vi "GUI - TDMS (V2.00).vi"(0 "Time Data IN":refnum<class "GSwFormDSP.lvclass">, 5 "error in (no error)":errorcluster, 7 "Application Name":string="GSwForm", 9 "State Queue":string[](array[string])=["SC >>> Initialize"], 11 "TDMS - READ":path, 13 "TDMS - WRITE":path) -> (12 "Loaded File":path, 14 "SubVI Time Data DUP":refnum<class "GSwFormDSP.lvclass">, 19 "error out":errorcluster)   [LabVIEW 2020, in "TDMS.lvclass"]
uses:
  TDMS.lvclass
  API/GSwFormDSP_class/GSwFormDSP.lvclass
  <vilib>/Utility/sysdir.llb/System Directory Type.ctl
  C:/Users/fcharett/docsWork/coding/20openSourceSPWB/API/Generic Utilities_class/Generic Utilities.lvclass
  <userlib>/_OpenG.lib/array/array.llb/Filter 1D Array with Scalar (String)__ogtk.vi
  <userlib>/_OpenG.lib/array/array.llb/Remove Duplicates from 1D Array (String)__ogtk.vi
  <vilib>/addons/_AddQ/G#Object/G#Object.lvclass
  API/Generic Utilities_class/Generic Utilities.lvclass
panel:
  in  "Task":T1(tab)
  in  "Import Signals":bool
  in  "Select Signal to Import":i32[](listbox)
  in  "Exit":bool
  in  "Downsampling":enum16{"None", "By 10", "By 100", "By 1000"}(ring)=enum."By 10"
  out "Base Folder":path
  out "Number of TDMS Files":i32
  in  "Select Base Folder":bool
  in  "Defrag ALL Files":bool
  in  "Channel List":i32[](listbox)
  in  "Refresh Signal Names":bool
  in  "Select Multi Files":bool
  out "File List":path[](array[path])
  out "group/channel names":string[][](array[string])
  out "All T0":timestamp[](array[timestamp])
  out "Valid T0":bool
  out "Time Data":waveform(dbl)[](graph)
  in  "READ - Select TDMS File":bool
  in  "WRITE - Select Wave File":bool
  out "State History":string[](array[string])
  out "State Index":i32
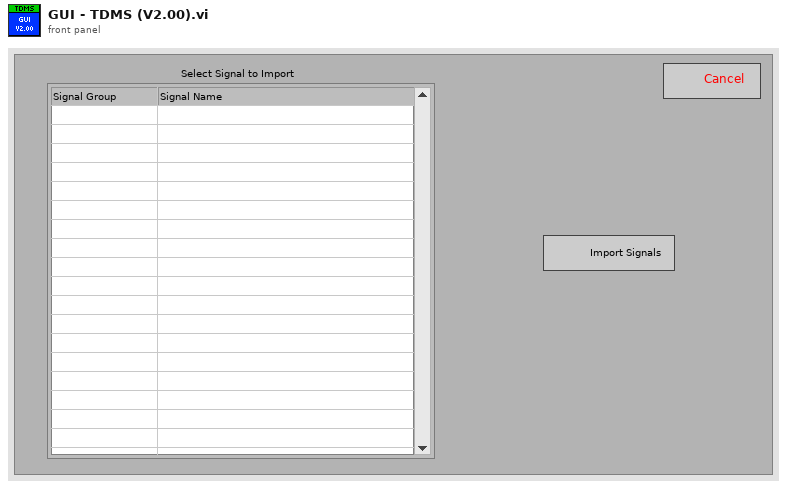
[diagram p1: front panel]
types:
  T1 = enum32{"TDMS Select Signal", "TDMS Folder", "Multi TDMS Files", "TDMS", "Settings"}
  T2 = enum32{"Invalid", "Standard", "Closed", "Hidden", "Minimized", "Maximized"}
  T3 = typedef "System Directory Type.ctl" = i32
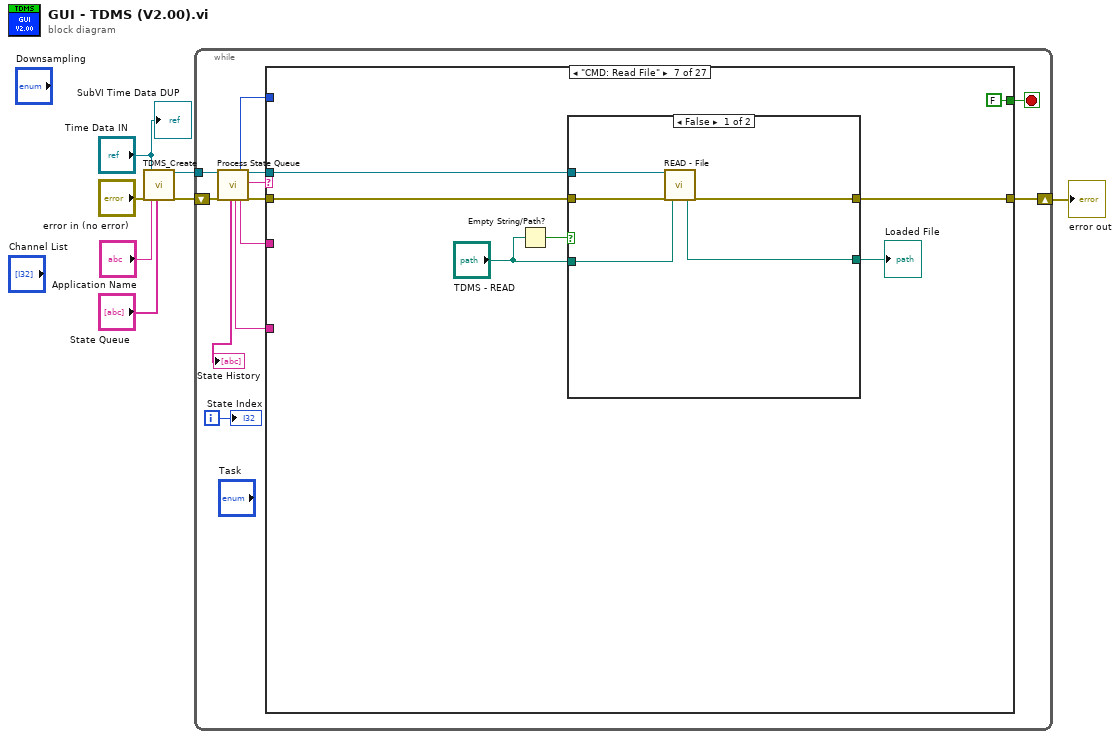
[diagram p0: block diagram]
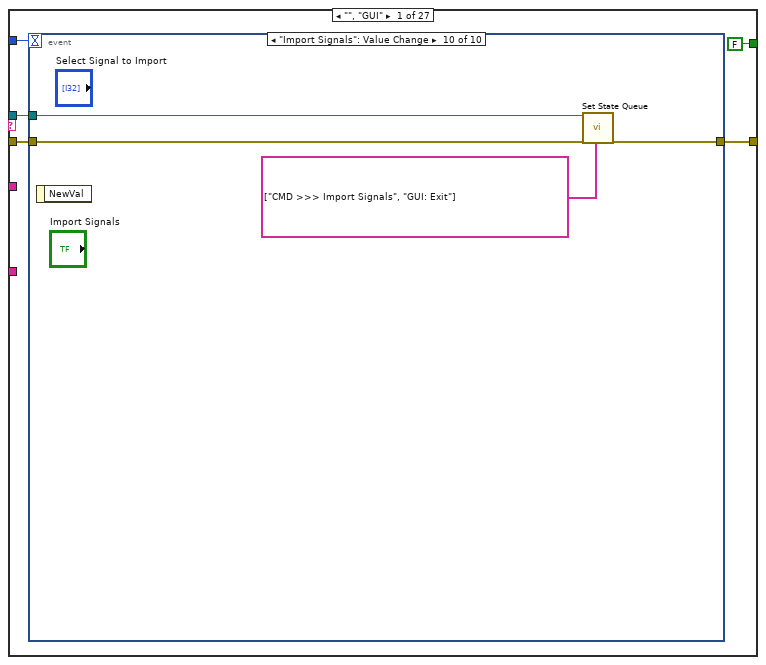
[diagram p2: hidden frame]
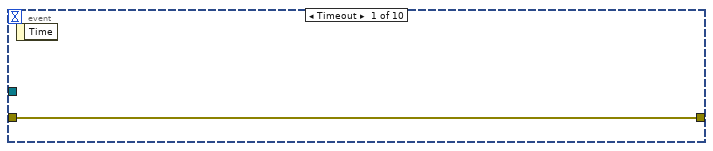
[diagram p3: hidden frame]
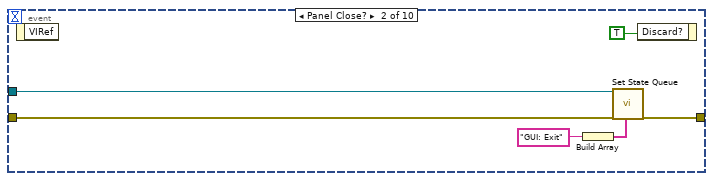
[diagram p4: hidden frame]
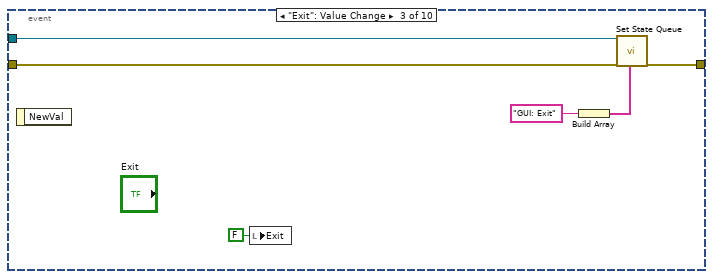
[diagram p5: hidden frame]
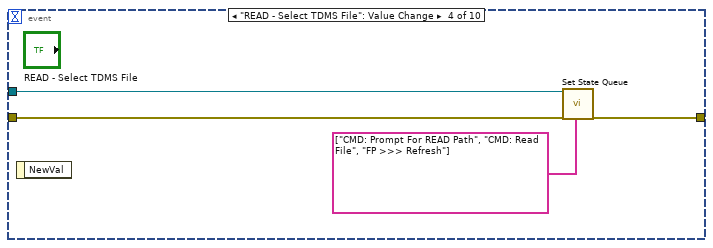
[diagram p6: hidden frame]
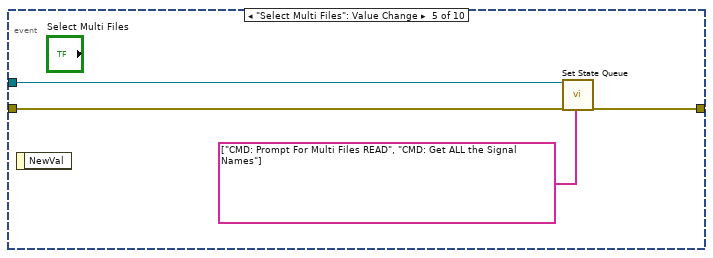
[diagram p7: hidden frame]
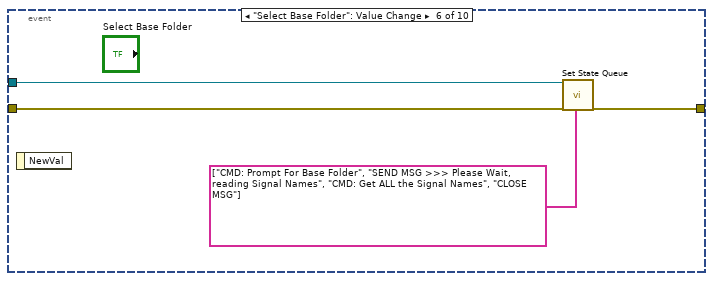
[diagram p8: hidden frame]
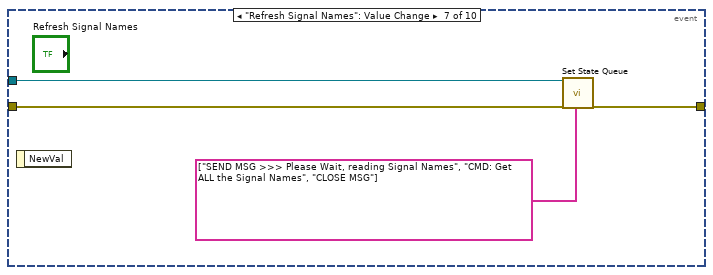
[diagram p9: hidden frame]
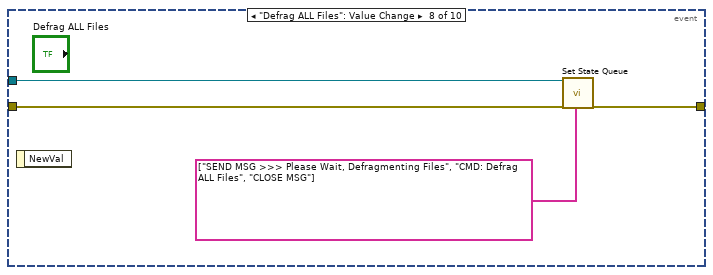
[diagram p10: hidden frame]
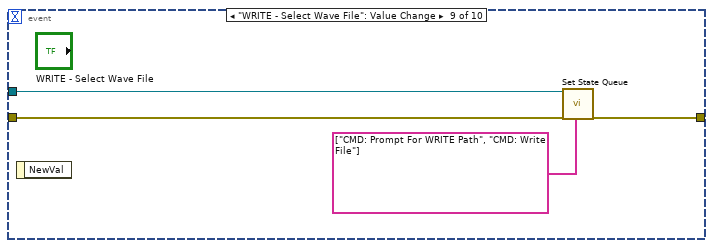
[diagram p11: hidden frame]
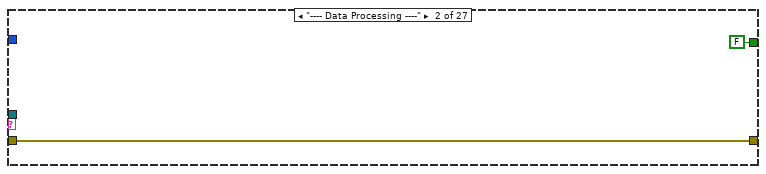
[diagram p12: hidden frame]
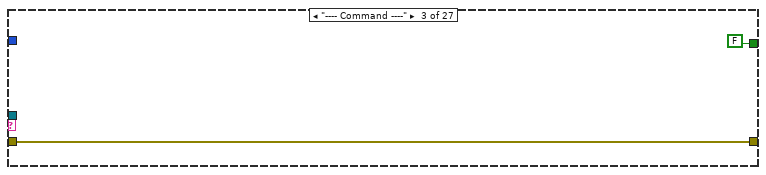
[diagram p13: hidden frame]
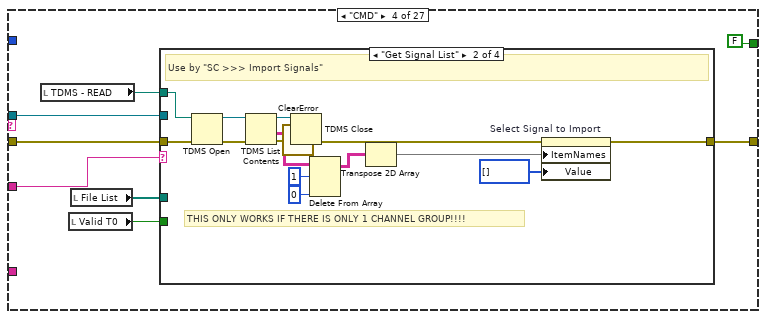
[diagram p14: hidden frame]
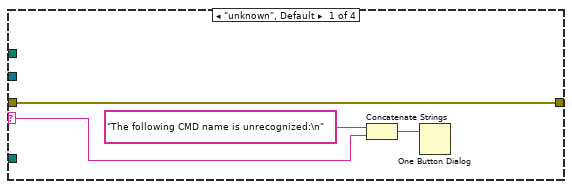
[diagram p15: hidden frame]
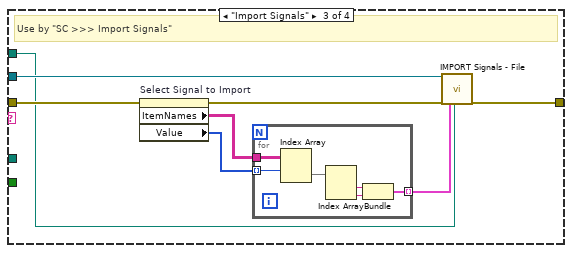
[diagram p16: hidden frame]
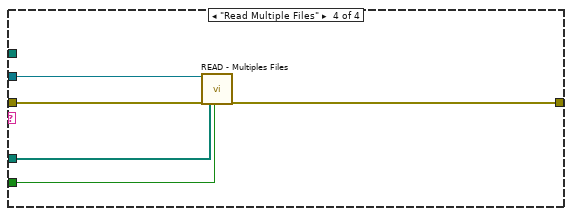
[diagram p17: hidden frame]
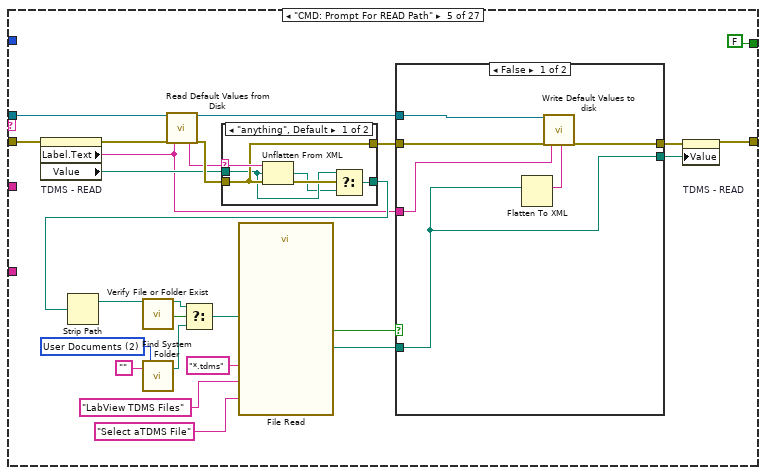
[diagram p18: hidden frame]
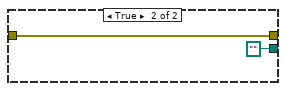
[diagram p19: hidden frame]
diagram:
  n1 = call "TDMS_Create.vi"("error in (no error)"="error in (no error)", "Time Data"="Time Data IN", "Application Name"="Application Name", "State Queue"="State Queue") -> ("reference out"=w7:refnum<class "TDMS.lvclass">, "error out"=w6:errorcluster)  [unwired: 14 in]
  n2 = while {
    shift-right: [w10] -> w2
    shift-left: w6 -> [w16]
    tunnel: w7 -> [w17]
    i -> [w18]
    stop <- w19 stop-if-true
    n3 = call "Process State Queue.vi"("reference in"=w17, "error in (no error)"=w16) -> ("State History"=→"State History":string[], "Additional Options"=w8:string, "Timeout"=w15:i32, "State Option"=w12:string, "reference out"=w14:refnum<class "TDMS.lvclass">, "Current State"=w13:string, "error out"=w11:errorcluster)  [unwired: 10 in, 1 out]
    n4 = case shown="\"CMD: Read File\"" w13 {
      selector: w13 -> [_ _ _ _ _ _ _ _ _ _ _ _ _ _ _ _ _ _ _ _ _ _ _ w614 _ _ _]
      tunnel: w14 -> [w22 _ _ w73 w140 w182 w205 w218 w250 w298 _ _ _ w404 _ w421 w476 _ w517 w538 w571 w596 _ _ _ _ w622]
      tunnel: [FALSE FALSE FALSE FALSE FALSE FALSE FALSE FALSE FALSE FALSE FALSE FALSE FALSE FALSE FALSE FALSE FALSE FALSE FALSE TRUE FALSE FALSE FALSE FALSE FALSE FALSE TRUE] -> w19
      tunnel: w15 -> [w23 _ _ _ _ _ _ _ _ _ _ _ _ _ _ _ _ _ _ _ _ _ _ _ _ _ _]
      tunnel: w12 -> [_ _ _ w76 _ _ _ _ _ _ _ _ _ w400 _ w422 w473 _ _ _ w580 _ _ _ _ _ _]
      tunnel: w11 -> [w21 w66 w68 w75 w139 w181 w204 w217 w249 w297 w339 w392 w397 w403 w416 w419 w475 w502 w514 w535 w570 w597 w610 w612 w617 w620 w623]
      tunnel: [w20 w66 w68 w74 w123 w165 w203 w216 w233 w283 w334 w389 w397 w402 w416 w420 w474 w502 w509 w534 w568 w593 w610 w612 errorcluster {"status"=FALSE, "code"=0, "source"=""} ("error out") w620 w624] -> w10
      tunnel: w8 -> [_ _ _ _ _ _ _ _ _ _ _ _ _ w399 _ w418 _ _ _ _ _ _ _ _ _ _ _]
      frame "", "GUI" {
        n5 = event shown="[9] \"Import Signals\": Value Change" {
          selector: _ -> [_ _ _ _ _ _ _ _ _ _]
          dyn-events: _ -> [_ _ _ _ _ _ _ _ _ _]
          timeout: w23 -> [_ _ _ _ _ _ _ _ _ _]
          tunnel: w22 -> [_ w29 w35 w40 w44 w48 w52 w56 w60 w64]
          tunnel: w21 -> [w25 w28 w33 w39 w43 w47 w51 w55 w59 w63]
          tunnel: [w25 w27 w34 w41 w45 w49 w53 w57 w61 w65] -> w20
          event Timeout {
            n6 = event-data() -> ()  [unwired: 1 in, 1 out]
          }
          event Panel Close? {
            n7 = event-data() -> ()  [unwired: 1 in, 1 out]
            n8 = Build Array("GUI: Exit") -> (w26:string[])
            n9 = call "Set State Queue.vi"("reference in"=w29, "error in (no error)"=w28, "State Queue"=w26) -> ("error out"=w27:errorcluster)  [unwired: 15 in, 1 out]
            n10 = event-data("Discard?"=TRUE) -> ()  [unwired: 1 in, 1 out]
          }
          event "Exit": Value Change {
            n11 = event-data() -> ()  [unwired: 1 in, 1 out]
            n12 = local write "Exit"(FALSE ("Exit")) -> ()
            n13 = Build Array("GUI: Exit") -> (w32:string[])
            n14 = call "Set State Queue.vi"("reference in"=w35, "error in (no error)"=w33, "State Queue"=w32) -> ("error out"=w34:errorcluster)  [unwired: 15 in, 1 out]
          }
          event "READ - Select TDMS File": Value Change {
            n15 = event-data() -> ()  [unwired: 1 in, 1 out]
            n16 = call "Set State Queue.vi"("reference in"=w40, "error in (no error)"=w39, "State Queue"=string[] ["CMD: Prompt For READ Path", "CMD: Read File", "FP >>> Refresh"]) -> ("error out"=w41:errorcluster)  [unwired: 15 in, 1 out]
          }
          event "Select Multi Files": Value Change {
            n17 = event-data() -> ()  [unwired: 1 in, 1 out]
            n18 = call "Set State Queue.vi"("reference in"=w44, "error in (no error)"=w43, "State Queue"=string[] ["CMD: Prompt For Multi Files READ", "CMD: Get ALL the Signal Names"]) -> ("error out"=w45:errorcluster)  [unwired: 15 in, 1 out]
          }
          event "Select Base Folder": Value Change {
            n19 = event-data() -> ()  [unwired: 1 in, 1 out]
            n20 = call "Set State Queue.vi"("reference in"=w48, "error in (no error)"=w47, "State Queue"=string[] ["CMD: Prompt For Base Folder", "SEND MSG >>> Please Wait, reading Signal Names", "CMD: Get ALL the Signal Names", "CLOSE MSG"]) -> ("error out"=w49:errorcluster)  [unwired: 15 in, 1 out]
          }
          event "Refresh Signal Names": Value Change {
            n21 = event-data() -> ()  [unwired: 1 in, 1 out]
            n22 = call "Set State Queue.vi"("reference in"=w52, "error in (no error)"=w51, "State Queue"=string[] ["SEND MSG >>> Please Wait, reading Signal Names", "CMD: Get ALL the Signal Names", "CLOSE MSG"]) -> ("error out"=w53:errorcluster)  [unwired: 15 in, 1 out]
          }
          event "Defrag ALL Files": Value Change {
            n23 = event-data() -> ()  [unwired: 1 in, 1 out]
            n24 = call "Set State Queue.vi"("reference in"=w56, "error in (no error)"=w55, "State Queue"=string[] ["SEND MSG >>> Please Wait, Defragmenting Files", "CMD: Defrag ALL Files", "CLOSE MSG"]) -> ("error out"=w57:errorcluster)  [unwired: 15 in, 1 out]
          }
          event "WRITE - Select Wave File": Value Change {
            n25 = event-data() -> ()  [unwired: 1 in, 1 out]
            n26 = call "Set State Queue.vi"("reference in"=w60, "error in (no error)"=w59, "State Queue"=string[] ["CMD: Prompt For WRITE Path", "CMD: Write File"]) -> ("error out"=w61:errorcluster)  [unwired: 15 in, 1 out]
          }
          event "Import Signals": Value Change {
            n27 = event-data() -> ()  [unwired: 1 in, 1 out]
            n28 = call "Set State Queue.vi"("reference in"=w64, "error in (no error)"=w63, "State Queue"=string[] ["CMD >>> Import Signals", "GUI: Exit"]) -> ("error out"=w65:errorcluster)  [unwired: 15 in, 1 out]
          }
        }
      }
      frame "---- Data Processing ----" {
      }
      frame "---- Command ----" {
      }
      frame "CMD" {
        n29 = local read "TDMS - READ"() -> (w72:path)
        n30 = local read "Valid T0"() -> (w70:bool)
        n31 = local read "File List"() -> (w71:path[])
        n32 = case shown="\"Get Signal List\"" w76 {
          selector: w76 -> [w79 _ _ _]
          tunnel: w75 -> [w78 w94 w102 w114]
          tunnel: [w78 w90 w103 w113] -> w74
          tunnel: w73 -> [_ _ w104 w115]
          tunnel: w72 -> [_ w83 w99 _]
          tunnel: w71 -> [_ _ _ w112]
          tunnel: w70 -> [_ _ _ w111]
          frame "unknown", Default {
            n33 = Concatenate Strings("The following CMD name is unrecognized:\n", w79) -> (w80:string)
            n34 = One Button Dialog(message=w80) -> ()  [unwired: 1 in, 1 out]
          }
          frame "Get Signal List" {
            # "THIS ONLY WORKS IF THERE IS ONLY 1 CHANNEL GROUP!!!!"
            # "Use by \"SC >>> Import Signals\""
            n35 = TDMS Open(8:w94, 11:w83) -> (0:w96:errorcluster, 3:w95:refnum<k34>)  [unwired: 5 in]
            n36 = TDMS List Contents(4:w96, 7:w95) -> (0:w82:errorcluster, 1:w88:string[][], 3:w92:refnum<k34>)  [unwired: 1 in, 1 out]
            n37 = call <vilib>:"ClearError.vi"("error in (no error)"=w82) -> ("error out"=w93:errorcluster)
            n38 = TDMS Close(8:w93, 11:w92) -> (0:w91:errorcluster)  [unwired: 1 out]
            n39 = Delete From Array(array=w88, length=1, index (col)=0 ("disabled index (col)")) -> (array with subset deleted=w85:string[][])  [unwired: 1 in, 1 out]
            n40 = Transpose 2D Array(2D array=w85) -> (transposed array=w89:string[][])
            n41 = property on="Select Signal to Import" class="MCListbox (strict)"(error in=w91, "ItemNames"=w89, "Value"=i32[] [] ("Select Signal to Import")) -> (error out=w90:errorcluster)  [unwired: 1 in, 1 out]
          }
          frame "Import Signals" {
            # "Use by \"SC >>> Import Signals\""
            n42 = property on="Select Signal to Import" class="MCListbox (strict)"(error in=w102) -> (error out=w98:errorcluster, "ItemNames"=w101:string[][], "Value"=w100:i32[])  [unwired: 1 in, 1 out]
            n43 = for {
              tunnel: w101 -> [w110]
              tunnel: w100 -> [w109] mode=indexing
              tunnel: [w105] -> w97 mode=indexing
              n44 = Index Array(array=w110, index (row)=w109) -> (element=w108:string[])  [unwired: 1 in]
              n45 = Index Array(array=w108) -> (element #1=w106:string, element #2=w107:string)  [unwired: 2 in]
              n46 = Bundle(w106, w107) -> (w105:cluster{string, string})  [unwired: 1 in]
            }
            n47 = call "IMPORT Signals - File.vi"("reference in"=w104, "error in (no error)"=w98, "Grp/Sig Names"=w97, "TDMS Path - READ"=w99) -> ("error out"=w103:errorcluster)  [unwired: 14 in, 1 out]
          }
          frame "Read Multiple Files" {
            n48 = call "READ - Multiples Files.vi"("reference in"=w115, "error in (no error)"=w114, "File List"=w112, "Valid T0"=w111) -> ("error out"=w113:errorcluster)  [unwired: 14 in, 1 out]
          }
        }
      }
      frame "CMD: Prompt For READ Path" {
        w130 = T3 2 items=["User Home"=0, "User Desktop"=1, "User Documents"=2, "User Application Data"=3, "User Preferences"=4, "User Temporary"=5, "Public Documents"=6, "Public Application Data"=7, "Public Preferences"=8, "Public Cache"=13, "System Core Libraries"=9, "System Installed Libraries"=10, "Application Files"=11, "Boot Volume Root"=12] ("system directory type")
        n49 = property on="TDMS - READ" class="Path"(error in=w139) -> (error out=w138:errorcluster, "Label.Text"=w118:string, "Value"=w136:path)  [unwired: 1 in, 1 out]
        n50 = call "Find System Folder.vi"("Application Name"="", "system directory type"=w130) -> ("System Folder"=w129:path)  [unwired: 16 in, 1 out]
        n51 = call-dynamic "Read Default Values from Disk.vi"("reference in"=w140, "error in (no error)"=w138, "Control Label"=w118) -> ("Value (XML String)"=w116:string, "reference out"=w119:refnum<class "TDMS.lvclass">, "error out"=w137:errorcluster)  [unwired: 14 in]
        n52 = case shown="\"anything\", Default" w116 {
          selector: w116 -> [w155 _]
          tunnel: [w150 w157] -> w135
          tunnel: w136 -> [w152 w157]
          tunnel: w137 -> [w153 w156]
          tunnel: [w153 w156] -> w121
          frame "anything", Default {
            n53 = Unflatten From XML(xml string=w155, type=w152, error in (no error)=w153) -> (value=w151:path, error out=w154:errorcluster)
            n54 = Select(t=w152, s=w154, f=w151) -> (s? t:f=w150:path)
          }
          frame "" {
            # "Either the file was not found or there was some error"
          }
        }
        n55 = Strip Path(path=w135) -> (stripped path=w134:path)  [unwired: 1 out]
        n56 = call "Verify File or Folder Exist.vi"("path"=w134) -> ("dup path"=w132:path, "file or folder exists?"=w133:bool)  [unwired: 16 in, 1 out]
        n57 = Select(t=w132, s=w133, f=w129) -> (s? t:f=w131:path)
        n58 = call "File Read"("start path"=w131, "button label"="Select aTDMS File", "pattern (all files)"="*.tdms", "pattern label"="LabView TDMS Files") -> ("selected path"=w117:path, "cancelled"=w124:bool)  [unwired: 8 in, 2 out]
        n59 = case shown="False" w124 {
          tunnel: [w143 w149] -> w122
          tunnel: w121 -> [w144 w149]
          tunnel: [w142 path ""] -> w120
          tunnel: w119 -> [w146 _]
          tunnel: w118 -> [w145 _]
          tunnel: w117 -> [w142 _]
          frame False {
            n60 = Flatten To XML(6:w142) -> (2:w147:string)
            n61 = call-dynamic "Write Default Values to disk.vi"("reference in"=w146, "error in (no error)"=w144, "Control Label"=w145, "Value (XML String)"=w147) -> ("error out"=w143:errorcluster)  [unwired: 14 in, 1 out]
          }
          frame True {
          }
        }
        n62 = property on="TDMS - READ" class="Path"(error in=w122, "Value"=w120) -> (error out=w123:errorcluster)  [unwired: 1 in, 1 out]
      }
      frame "CMD: Prompt For WRITE Path" {
        w172 = T3 2 items=["User Home"=0, "User Desktop"=1, "User Documents"=2, "User Application Data"=3, "User Preferences"=4, "User Temporary"=5, "Public Documents"=6, "Public Application Data"=7, "Public Preferences"=8, "Public Cache"=13, "System Core Libraries"=9, "System Installed Libraries"=10, "Application Files"=11, "Boot Volume Root"=12] ("system directory type")
        n63 = property on="TDMS - WRITE" class="Path"(error in=w181) -> (error out=w180:errorcluster, "Label.Text"=w160:string, "Value"=w178:path)  [unwired: 1 in, 1 out]
        n64 = call "Find System Folder.vi"("Application Name"="", "system directory type"=w172) -> ("System Folder"=w171:path)  [unwired: 16 in, 1 out]
        n65 = call-dynamic "Read Default Values from Disk.vi"("reference in"=w182, "error in (no error)"=w180, "Control Label"=w160) -> ("Value (XML String)"=w158:string, "reference out"=w161:refnum<class "TDMS.lvclass">, "error out"=w179:errorcluster)  [unwired: 14 in]
        n66 = case shown="\"anything\", Default" w158 {
          selector: w158 -> [w197 _]
          tunnel: [w192 w199] -> w177
          tunnel: w178 -> [w194 w199]
          tunnel: w179 -> [w195 w198]
          tunnel: [w195 w198] -> w163
          frame "anything", Default {
            n67 = Unflatten From XML(xml string=w197, type=w194, error in (no error)=w195) -> (value=w193:path, error out=w196:errorcluster)
            n68 = Select(t=w194, s=w196, f=w193) -> (s? t:f=w192:path)
          }
          frame "" {
            # "Either the file was not found or there was some error"
          }
        }
        n69 = Strip Path(path=w177) -> (stripped path=w176:path)  [unwired: 1 out]
        n70 = call "Verify File or Folder Exist.vi"("path"=w176) -> ("dup path"=w174:path, "file or folder exists?"=w175:bool)  [unwired: 16 in, 1 out]
        n71 = Select(t=w174, s=w175, f=w171) -> (s? t:f=w173:path)
        n72 = call "File Write"("start path"=w173, "button label"="Select aTDMS File", "pattern (all files)"="*.tdms", "pattern label"="LabView TDMS Files") -> ("selected path"=w159:path, "cancelled"=w166:bool)  [unwired: 8 in, 2 out]
        n73 = case shown="False" w166 {
          tunnel: [w185 w191] -> w164
          tunnel: w163 -> [w186 w191]
          tunnel: [w184 path ""] -> w162
          tunnel: w161 -> [w188 _]
          tunnel: w160 -> [w187 _]
          tunnel: w159 -> [w184 _]
          frame False {
            n74 = Flatten To XML(6:w184) -> (2:w189:string)
            n75 = call-dynamic "Write Default Values to disk.vi"("reference in"=w188, "error in (no error)"=w186, "Control Label"=w187, "Value (XML String)"=w189) -> ("error out"=w185:errorcluster)  [unwired: 14 in, 1 out]
          }
          frame True {
          }
        }
        n76 = property on="TDMS - WRITE" class="Path"(error in=w164, "Value"=w162) -> (error out=w165:errorcluster)  [unwired: 1 in, 1 out]
      }
      frame "CMD: Read File" {
        n77 = Empty String/Path?(string/path="TDMS - READ") -> (empty?=w202:bool)
        n78 = case shown="False" w202 {
          tunnel: w205 -> [w211 _]
          tunnel: w204 -> [w210 w213]
          tunnel: [w208 w213] -> w203
          tunnel: "TDMS - READ" -> [w209 _]
          tunnel: [w207 path ""] -> w200
          frame False {
            n79 = call "READ - File.vi"("reference in"=w211, "error in (no error)"=w210, "TDMS Path - READ"=w209) -> ("File Loaded"=w207:path, "error out"=w208:errorcluster)  [unwired: 14 in, 1 out]
          }
          frame True {
            # "User cancelled, so do nothing!"
          }
        }
        "Loaded File" <- w200
      }
      frame "CMD: Write File" {
        n80 = Empty String/Path?(string/path="TDMS - WRITE") -> (empty?=w215:bool)
        n81 = case shown="False" w215 {
          tunnel: w218 -> [w223 _]
          tunnel: w217 -> [w222 w224]
          tunnel: [w220 w224] -> w216
          tunnel: "TDMS - WRITE" -> [w221 _]
          frame False {
            n82 = call "WRITE - File.vi"("reference in"=w223, "error in (no error)"=w222, "TDMS Path - WRITE"=w221) -> ("error out"=w220:errorcluster)  [unwired: 15 in, 1 out]
          }
          frame True {
            # "User cancelled, so do nothing!"
          }
        }
      }
      frame "CMD: Prompt For Multi Files READ" {
        w240 = T3 2 items=["User Home"=0, "User Desktop"=1, "User Documents"=2, "User Application Data"=3, "User Preferences"=4, "User Temporary"=5, "Public Documents"=6, "Public Application Data"=7, "Public Preferences"=8, "Public Cache"=13, "System Core Libraries"=9, "System Installed Libraries"=10, "Application Files"=11, "Boot Volume Root"=12] ("system directory type")
        n83 = property on="TDMS - READ" class="Path"(error in=w249) -> (error out=w248:errorcluster, "Label.Text"=w228:string, "Value"=w246:path)  [unwired: 1 in, 1 out]
        n84 = call "Find System Folder.vi"("Application Name"="", "system directory type"=w240) -> ("System Folder"=w239:path)  [unwired: 16 in, 1 out]
        n85 = call-dynamic "Read Default Values from Disk.vi"("reference in"=w250, "error in (no error)"=w248, "Control Label"=w228) -> ("Value (XML String)"=w225:string, "reference out"=w229:refnum<class "TDMS.lvclass">, "error out"=w247:errorcluster)  [unwired: 14 in]
        n86 = case shown="\"anything\", Default" w225 {
          selector: w225 -> [w271 _]
          tunnel: [w266 w273] -> w245
          tunnel: w246 -> [w268 w273]
          tunnel: w247 -> [w269 w272]
          tunnel: [w269 w272] -> w231
          frame "anything", Default {
            n87 = Unflatten From XML(xml string=w271, type=w268, error in (no error)=w269) -> (value=w267:path, error out=w270:errorcluster)
            n88 = Select(t=w268, s=w270, f=w267) -> (s? t:f=w266:path)
          }
          frame "" {
            # "Either the file was not found or there was some error"
          }
        }
        n89 = Strip Path(path=w245) -> (stripped path=w244:path)  [unwired: 1 out]
        n90 = call "Verify File or Folder Exist.vi"("path"=w244) -> ("dup path"=w242:path, "file or folder exists?"=w243:bool)  [unwired: 16 in, 1 out]
        n91 = Select(t=w242, s=w243, f=w239) -> (s? t:f=w241:path)
        n92 = call "Multi Files Read"("start path"=w241, "button label"="Select aTDMS File", "pattern (all files)"="*.tdms", "pattern label"="LabView TDMS Files") -> ("selected paths"=w227:path[], "cancelled"=w234:bool)  [unwired: 8 in, 2 out]
        n93 = case shown="False" w234 {
          tunnel: [w254 w259] -> w232
          tunnel: w231 -> [w255 w262]
          tunnel: [w253 path ""] -> w230
          tunnel: w229 -> [w257 w263]
          tunnel: w228 -> [w256 _]
          tunnel: w227 -> [w252 _]
          tunnel: [w252 path[] [] ("selected paths")] -> w226
          frame False {
            # "Just to save default path"
            n94 = Index Array(array=w252) -> (element=w253:path)  [unwired: 1 in]
            n95 = Flatten To XML(6:w253) -> (2:w258:string)
            n96 = call-dynamic "Write Default Values to disk.vi"("reference in"=w257, "error in (no error)"=w255, "Control Label"=w256, "Value (XML String)"=w258) -> ("error out"=w254:errorcluster)  [unwired: 14 in, 1 out]
          }
          frame True {
            # "User cancelled, so abort the queue"
            n97 = call "Set State Queue.vi"("reference in"=w263, "error in (no error)"=w262, "State Queue Options"=enum16{"Replace", "Append", "Prepend"}."Replace", "State Queue"=string[] []) -> ("error out"=w259:errorcluster)  [unwired: 14 in, 1 out]
          }
        }
        "File List" <- w226
        n98 = property on="TDMS - READ" class="Path"(error in=w232, "Value"=w230) -> (error out=w233:errorcluster)  [unwired: 1 in, 1 out]
      }
      frame "CMD: Prompt For Base Folder" {
        w288 = T3 2 items=["User Home"=0, "User Desktop"=1, "User Documents"=2, "User Application Data"=3, "User Preferences"=4, "User Temporary"=5, "Public Documents"=6, "Public Application Data"=7, "Public Preferences"=8, "Public Cache"=13, "System Core Libraries"=9, "System Installed Libraries"=10, "Application Files"=11, "Boot Volume Root"=12] ("system directory type")
        n99 = property on="TDMS - READ" class="Path"(error in=w297) -> (error out=w296:errorcluster, "Label.Text"=w278:string, "Value"=w294:path)  [unwired: 1 in, 1 out]
        n100 = call "Find System Folder.vi"("Application Name"="", "system directory type"=w288) -> ("System Folder"=w287:path)  [unwired: 16 in, 1 out]
        n101 = call-dynamic "Read Default Values from Disk.vi"("reference in"=w298, "error in (no error)"=w296, "Control Label"=w278) -> ("Value (XML String)"=w274:string, "reference out"=w279:refnum<class "TDMS.lvclass">, "error out"=w295:errorcluster)  [unwired: 14 in]
        n102 = case shown="\"anything\", Default" w274 {
          selector: w274 -> [w323 _]
          tunnel: [w318 w325] -> w293
          tunnel: w294 -> [w320 w325]
          tunnel: w295 -> [w321 w324]
          tunnel: [w321 w324] -> w281
          frame "anything", Default {
            n103 = Unflatten From XML(xml string=w323, type=w320, error in (no error)=w321) -> (value=w319:path, error out=w322:errorcluster)
            n104 = Select(t=w320, s=w322, f=w319) -> (s? t:f=w318:path)
          }
          frame "" {
            # "Either the file was not found or there was some error"
          }
        }
        n105 = Strip Path(path=w293) -> (stripped path=w292:path)  [unwired: 1 out]
        n106 = call "Verify File or Folder Exist.vi"("path"=w292) -> ("dup path"=w290:path, "file or folder exists?"=w291:bool)  [unwired: 16 in, 1 out]
        n107 = Select(t=w290, s=w291, f=w287) -> (s? t:f=w289:path)
        n108 = call "Select Base Folder"("start path"=w289, "button label"="Select a Folder") -> ("selected path"=w277:path, "cancelled"=w284:bool)  [unwired: 10 in, 2 out]
        n109 = case shown="False" w284 {
          tunnel: [w306 w312] -> w282
          tunnel: w281 -> [w307 w315]
          tunnel: [w304 w311] -> w280
          tunnel: w279 -> [w309 w316]
          tunnel: w278 -> [w308 _]
          tunnel: w277 -> [w300 _]
          tunnel: [w302 path[] [] ("selected paths")] -> w276
          tunnel: [w300 w311] -> w275
          frame False {
            # "Just to save default path"
            n110 = call <vilib>:"Recursive File List.vi"("pattern"="*.tdms", "Folder Path"=w300) -> ("Number of Files"=→"Number of TDMS Files":i32, "All Files in Dir"=w302:path[])  [unwired: 5 in, 3 out]
            n111 = Build Path(base path=w300, name or relative path="Base Folder.tdms") -> (appended path=w304:path)
            n112 = Flatten To XML(6:w304) -> (2:w310:string)
            n113 = call-dynamic "Write Default Values to disk.vi"("reference in"=w309, "error in (no error)"=w307, "Control Label"=w308, "Value (XML String)"=w310) -> ("error out"=w306:errorcluster)  [unwired: 14 in, 1 out]
          }
          frame True {
            w311 = path ""
            # "User cancelled, so abort the queue"
            n114 = call "Set State Queue.vi"("reference in"=w316, "error in (no error)"=w315, "State Queue Options"=enum16{"Replace", "Append", "Prepend"}."Replace", "State Queue"=string[] []) -> ("error out"=w312:errorcluster)  [unwired: 14 in, 1 out]
          }
        }
        "Base Folder" <- w275
        n115 = property on="TDMS - READ" class="Path"(error in=w282, "Value"=w280) -> (error out=w283:errorcluster)  [unwired: 1 in, 1 out]
        n116 = local write "File List"(w276) -> ()
      }
      frame "CMD: Get ALL the Signal Names" {
        n117 = property on="File List" class="Arr (strict)"(error in=w339) -> (error out=w338:errorcluster, "Value"=w337:path[])  [unwired: 1 in, 1 out]
        n118 = for {
          shift-right: [w360] -> w335
          shift-left: w338 -> [w362]
          tunnel: w337 -> [w358] mode=indexing
          shift-right: [w356] -> w333
          shift-left: string[] [] -> [w355]
          shift-right: [w344] -> w330
          shift-left: timestamp[] [] -> [w345]
          tunnel: timestamp(0 s since 1904-01-01) -> [w347]
          tunnel: "wf_start_time" ("property name") -> [w346]
          n119 = TDMS Open(8:w362, 11:w358) -> (0:w361:errorcluster, 3:w359:refnum<k34>)  [unwired: 5 in]
          n120 = TDMS List Contents(4:w361, 7:w359) -> (0:w341:errorcluster, 1:w342:string[][], 3:w350:refnum<k34>)  [unwired: 1 in, 1 out]
          "group/channel names" <- w342
          n121 = Transpose 2D Array(2D array=w342) -> (transposed array=w343:string[][])
          n122 = call <vilib>:"ClearError.vi"("error in (no error)"=w341) -> ("error out"=w351:errorcluster)
          n123 = for {
            shift-right: [w372] -> w348
            shift-left: w351 -> [w373]
            shift-right: [w371] -> w349
            shift-left: w350 -> [w374]
            tunnel: w347 -> [w370]
            tunnel: w346 -> [w369]
            shift-right: [w365] -> w344
            shift-left: w345 -> [w366]
            tunnel: w343 -> [w368] mode=indexing
            n124 = Index Array(array=w368) -> (element #1=w367:string, element #2=w364:string)  [unwired: 2 in]
            n125 = Empty String/Path?(string/path=w364) -> (empty?=w363:bool)
            n126 = case shown="False" w363 {
              tunnel: w374 -> [w385 w388]
              tunnel: w373 -> [w384 w387]
              tunnel: [w383 w387] -> w372
              tunnel: [w382 w388] -> w371
              tunnel: w370 -> [w381 _]
              tunnel: w369 -> [w380 _]
              tunnel: w367 -> [w379 _]
              tunnel: w366 -> [w378 w386]
              tunnel: [w377 w386] -> w365
              tunnel: w364 -> [w375 _]
              frame False {
                n127 = TDMS Get Properties(5:w381, 7:w380, 8:w384, 9:w375, 10:w379, 11:w385) -> (0:w383:errorcluster, 3:w382:refnum<k34>, 4:w376:timestamp)  [unwired: 3 out]
                n128 = Build Array (concatenate)(w378, w376) -> (w377:timestamp[])
              }
              frame True {
              }
            }
          }
          n129 = Index Array(array=w342, index (row)=1) -> (element=w354:string[])  [unwired: 1 in]
          n130 = call-poly <userlib>:"Filter 1D Array__ogtk.vi"("items to filter"="", "array"=w354) -> ("filtered array"=w353:string[])  [unwired: 4 in, 1 out]
          n131 = Build Array (concatenate)(w355, w353) -> (w356:string[])
          n132 = TDMS Close(8:w348, 11:w349) -> (0:w360:errorcluster)  [unwired: 1 out]
        }
        "All T0" <- w330
        n133 = Not Equal To 0?(x=w330) -> (x != 0?=w329:bool[])
        n134 = And Array Elements(Boolean array=w329) -> (logical AND=→"Valid T0":bool)
        n135 = call-poly <userlib>:"Remove Duplicates from 1D Array__ogtk.vi"("Input Array"=w333) -> ("Output Array"=w332:string[])  [unwired: 1 out]
        n136 = property on="Channel List" class="LstBox (strict)"(error in=w335, "Item Names"=w332) -> (error out=w334:errorcluster)  [unwired: 1 in, 1 out]
      }
      frame "CMD: Defrag ALL Files" {
        n137 = property on="File List" class="Arr (strict)"(error in=w392) -> (error out=w391:errorcluster, "Value"=w390:path[])  [unwired: 1 in, 1 out]
        n138 = for {
          shift-right: [w394] -> w389
          shift-left: w391 -> [w395]
          tunnel: w390 -> [w396] mode=indexing
          n139 = TDMS Defragment(4:w395, 7:w396) -> (0:w394:errorcluster)
        }
      }
      frame "---- Scripts ----" {
      }
      frame "SC" {
        (unwired) string[] ["GUI: Initialize Ref", "CMD: Prompt For Multi Files READ", "CTRL >>> Verify - READ File Path", "CMD: Get ALL the Signal Names", "CMD >>> Read Multiple Files", "CTRL >>> Task Tab >> Import Signals", "CMD >>> Get Signal List", "FP >>> Open"] ("State Queue OUT")
        n140 = case shown="\"Import Signals\"" w400 {
          selector: w400 -> [w407 _ _ _]
          tunnel: [string[] [] ("State Queue OUT") string[] ["GUI: Initialize Ref", "CTRL >>> Base Folder", "CTRL >>> Nb TDMS Files", "CTRL >>> Channel List", "CTRL >>> File Path List", "FP >>> Open"] ("State Queue OUT") w412 string[] ["CMD: Prompt For Multi Files READ", "CTRL >>> Verify - READ File Path", "CMD: Get ALL the Signal Names", "CMD >>> Read Multiple Files", "Quit"] ("State Queue OUT")] -> w401
          tunnel: w399 -> [_ _ w411 _]
          frame "False", Default {
            n141 = Concatenate Strings("The following SC name is unrecognized:\n", w407) -> (w408:string)
            n142 = One Button Dialog(message=w408) -> ()  [unwired: 1 in, 1 out]
          }
          frame "Initialize" {
          }
          frame "Import Signals" {
            n143 = case shown="\"Single Channel\"" w411 {
              tunnel: [string[] ["GUI: Initialize Ref", "CMD: Prompt For READ Path", "CTRL >>> Verify - READ File Path", "CTRL >>> Task Tab >> Import Signals", "CMD >>> Get Signal List", "CTRL >>> Import Signal >> Select 1 or More", "FP >>> Open"] ("State Queue OUT") string[] ["GUI: Initialize Ref", "CMD: Prompt For READ Path", "CTRL >>> Verify - READ File Path", "CTRL >>> Task Tab >> Import Signals", "CMD >>> Get Signal List", "CTRL >>> Import Signal >> Limit selection to 1", "FP >>> Open"] ("State Queue OUT")] -> w412
              frame "", Default {
              }
              frame "Single Channel" {
              }
            }
          }
          frame "Multiple Files" {
            # "This Step verify if ALL the channels T0 are valid!"
          }
        }
        n144 = call "Set State Queue.vi"("reference in"=w404, "error in (no error)"=w403, "State Queue"=w401) -> ("error out"=w402:errorcluster)  [unwired: 15 in, 1 out]
      }
      frame "---- Front Panel Mgmt ----" {
      }
      frame "CTRL" {
        n145 = case shown="\"Import Signal\"" w422 {
          selector: w422 -> [w424 _ _ _ _ _ _ _]
          tunnel: w421 -> [_ _ _ _ _ _ w448 _]
          tunnel: [w425 w429 w439 w441 w443 w446 w450 w461] -> w420
          tunnel: w419 -> [w425 w428 w440 w442 w444 w447 w449 w460]
          tunnel: w418 -> [_ w430 _ _ _ _ _ w462]
          frame "unknown", Default {
            n146 = Concatenate Strings("The following control name is unrecognized:\n", w424) -> (w426:string)
            n147 = One Button Dialog(message=w426) -> ()  [unwired: 1 in, 1 out]
          }
          frame "Task Tab" {
            n148 = case shown="\"unknown\", Default" w430 {
              selector: w430 -> [w432 _]
              tunnel: [w431 w437] -> w429
              tunnel: w428 -> [w431 w438]
              frame "unknown", Default {
                n149 = Concatenate Strings("The following \"CTRL >>> Task Tab\" name is unrecognized:\n", w432) -> (w433:string)
                n150 = One Button Dialog(message=w433) -> ()  [unwired: 1 in, 1 out]
              }
              frame "Import Signals" {
                n151 = property on="Task" class="TabCtl (strict)"(error in=w438, "Value"=T1."TDMS Select Signal" ("Task"), "PageSelVis"=FALSE ("Page Selector Visible")) -> (error out=w437:errorcluster)  [unwired: 1 in, 1 out]
              }
            }
          }
          frame "Base Folder" {
            n152 = invoke on="Base Folder" class="Path" method="Reinit To Default"(error in=w440) -> (error out=w439:errorcluster)  [unwired: 2 in, 2 out]
          }
          frame "Nb TDMS Files" {
            n153 = invoke on="Number of TDMS Files" class="DigNum (strict)" method="Reinit To Default"(error in=w442) -> (error out=w441:errorcluster)  [unwired: 2 in, 2 out]
          }
          frame "File Path List" {
            n154 = invoke on="File List" class="Arr (strict)" method="Reinit To Default"(error in=w444) -> (error out=w443:errorcluster)  [unwired: 2 in, 2 out]
          }
          frame "Channel List" {
            n155 = property on="Channel List" class="LstBox (strict)"(error in=w447, "Item Names"=string[] []) -> (error out=w446:errorcluster)  [unwired: 1 in, 1 out]
          }
          frame "Verify - READ File Path" {
            # "This is used by \"SC >>> Import Signals\""
            n156 = local read "TDMS - READ"() -> (w452:path)
            n157 = call "Verify File or Folder Exist.vi"("path"=w452) -> ("file or folder exists?"=w451:bool)  [unwired: 16 in, 2 out]
            n158 = case shown="False" w451 {
              tunnel: [w453 w459] -> w450
              tunnel: w449 -> [w455 w459]
              tunnel: w448 -> [w454 _]
              frame False {
                # "There are NO file, so exit the interface."
                n159 = Build Array("GUI: Exit") -> (w457:string[])
                n160 = call "Set State Queue.vi"("reference in"=w454, "error in (no error)"=w455, "State Queue Options"=enum16{"Replace", "Append", "Prepend"}."Replace", "State Queue"=w457) -> ("error out"=w453:errorcluster)  [unwired: 14 in, 1 out]
              }
              frame True {
                # "The File is available, so do nothing!"
              }
            }
          }
          frame "Import Signal" {
            n161 = case shown="\"Select 1 or More\"" w462 {
              selector: w462 -> [w464 _ _]
              tunnel: [w463 w467 w470] -> w461
              tunnel: w460 -> [w463 w469 w472]
              frame "False", Default {
                n162 = Concatenate Strings("The following \"CTRL >>> Import Signal\" name is unrecognized:\n", w464) -> (w465:string)
                n163 = One Button Dialog(message=w465) -> ()  [unwired: 1 in, 1 out]
              }
              frame "Limit selection to 1" {
                n164 = property on="Select Signal to Import" class="MCListbox (strict)"(error in=w469, "SelMode"=1 ("Selection Mode")) -> (error out=w467:errorcluster)  [unwired: 1 in, 1 out]
              }
              frame "Select 1 or More" {
                n165 = property on="Select Signal to Import" class="MCListbox (strict)"(error in=w472, "SelMode"=3 ("Selection Mode")) -> (error out=w470:errorcluster)  [unwired: 1 in, 1 out]
              }
            }
          }
        }
      }
      frame "FP" {
        n166 = case shown="\"Refresh\"" w473 {
          selector: w473 -> [w479 _ _]
          tunnel: w476 -> [_ w486 w499]
          tunnel: w475 -> [w478 w485 w498]
          tunnel: [w478 w482 w496] -> w474
          frame "", Default {
            n167 = Concatenate Strings("The following FP is unrecognized:\n", w479) -> (w480:string)
            n168 = One Button Dialog(message=w480) -> ()  [unwired: 1 in, 1 out]
          }
          frame "Open" {
            n169 = call-dynamic "Get VI Ref.vi"("reference in"=w486, "error in (no error)"=w485) -> ("GUI VI Ref"=w483:refnum<vi>, "error out"=w484:errorcluster)  [unwired: 14 in, 2 out]
            n170 = property class="VI"(reference=w483, error in=w484) -> (reference out=w488:refnum<vi>, error out=w489:errorcluster, "Front Panel.Open"=w487:bool)
            n171 = case shown="False" w487 {
              tunnel: [w492 w495] -> w482
              tunnel: w489 -> [w491 w495]
              tunnel: w488 -> [w490 _]
              frame False {
                n172 = invoke class="VI" method="FP.Open"(reference=w490, error in=w491, "Activate"=TRUE, "State"=T2."Standard") -> (error out=w492:errorcluster)  [unwired: 1 in, 4 out]
              }
              frame True {
              }
            }
          }
          frame "Refresh" {
            n173 = call "Get - Time Data OBJ.vi"("reference in"=w499, "error in (no error)"=w498) -> ("Time Data OBJ"=w501:refnum<class "GSwFormDSP.lvclass">, "error out"=w500:errorcluster)  [unwired: 15 in, 1 out]
            n174 = call-dynamic "Get - wForms.vi"("reference in"=w501, "error in (no error)"=w500) -> ("wForms"=→"Time Data":waveform(dbl)[], "error out"=w496:errorcluster)  [unwired: 14 in, 2 out]
          }
        }
      }
      frame "---- GUI Functions ----" {
      }
      frame "GUI: Initialize Ref" {
        n175 = control-ref of="GUI Reference"() -> (w513:refnum<vi>)
        n176 = call "Set VI Ref.vi"("reference in"=w517, "error in (no error)"=w514, "ReInit All to Default?"=FALSE, "GUI VI Ref"=w513) -> ("reference out"=w516:refnum<class "TDMS.lvclass">, "error out"=w512:errorcluster)  [unwired: 14 in]
        n177 = call "Set Close Panel (Yes or No).vi"("reference in"=w516, "error in (no error)"=w512) -> ("reference out"=w515:refnum<class "TDMS.lvclass">, "error out"=w511:errorcluster)  [unwired: 16 in]
        n178 = call "Set Message Window Ref.vi"("reference in"=w515, "error in (no error)"=w511) -> ("reference out"=w508:refnum<class "TDMS.lvclass">, "error out"=w507:errorcluster)  [unwired: 16 in]
        n179 = call "Get - Time Data OBJ State.vi"("reference in"=w508, "error in (no error)"=w507) -> ("New Time Data Obj?"=w504:bool, "reference out"=w505:refnum<class "TDMS.lvclass">, "error out"=w506:errorcluster)  [unwired: 15 in]
        n180 = case shown="True" w504 {
          tunnel: [w519 w522] -> w509
          tunnel: w506 -> [w519 w521]
          tunnel: w505 -> [_ w520]
          frame False {
          }
          frame True {
            n181 = call "Get - Time Data OBJ.vi"("reference in"=w520, "error in (no error)"=w521) -> ("Time Data OBJ"=w524:refnum<class "GSwFormDSP.lvclass">, "error out"=w523:errorcluster)  [unwired: 15 in, 1 out]
            n182 = call "Set - wForms.vi"("reference in"=w524, "error in (no error)"=w523, "Init wForms"=TRUE) -> ("error out"=w522:errorcluster)  [unwired: 15 in, 1 out]
          }
        }
      }
      frame "GUI: Exit" {
        n183 = call-dynamic "Get Message Window Ref.vi"("reference in"=w538, "error in (no error)"=w535) -> ("reference out"=w537:refnum<class "TDMS.lvclass">, "Msg Win Ref"=w533:refnum<vi>, "error out"=w536:errorcluster)  [unwired: 15 in]
        n184 = call-dynamic "Get VI Ref.vi"("reference in"=w537, "error in (no error)"=w536) -> ("reference out"=w542:refnum<class "TDMS.lvclass">, "GUI VI Ref"=w540:refnum<vi>, "error out"=w541:errorcluster)  [unwired: 14 in, 1 out]
        n185 = call-dynamic "Get Close Panel (Yes or No).vi"("reference in"=w542, "error in (no error)"=w541) -> ("Close Panel?"=w543:bool, "reference out"=w532:refnum<class "TDMS.lvclass">, "error out"=w530:errorcluster)  [unwired: 15 in]
        n186 = call "Get - Time Data OBJ State.vi"("reference in"=w532, "error in (no error)"=w530) -> ("New Time Data Obj?"=w528:bool, "reference out"=w531:refnum<class "TDMS.lvclass">, "error out"=w529:errorcluster)  [unwired: 15 in]
        n187 = call-dynamic "Destroy.vi"("reference in"=w531, "error in (no error)"=w529) -> ("error out"=w547:errorcluster)  [unwired: 16 in, 1 out]
        n188 = case shown="False" w528 {
          tunnel: w547 -> [w549 w551]
          tunnel: [w549 w550] -> w539
          frame False {
          }
          frame True {
            n189 = call <vilib>:"GarbageCollector.vi"("error in (no error)"=w551) -> ("error out"=w550:errorcluster)  [unwired: 16 in, 2 out]
          }
        }
        n190 = Close Reference(reference=w533, error in (no error)=w539) -> (error out=w546:errorcluster)
        n191 = case shown="False" w543 {
          tunnel: w546 -> [w553 w557]
          tunnel: [w553 w556] -> w544
          tunnel: [w552 w555] -> w545
          tunnel: w540 -> [w552 w554]
          frame False {
          }
          frame True {
            n192 = property class="VI"(reference=w554, error in=w557) -> (reference out=w559:refnum<vi>, error out=w558:errorcluster, "Front Panel.Open"=w560:bool)
            n193 = case shown="True" w560 {
              tunnel: [w562 w566] -> w556
              tunnel: w558 -> [w562 w565]
              tunnel: w559 -> [w561 w564]
              tunnel: [w561 w563] -> w555
              frame False {
              }
              frame True {
                n194 = invoke class="VI" method="FP.Close"(reference=w564, error in=w565) -> (reference out=w563:refnum<vi>, error out=w566:errorcluster)  [unwired: 1 in, 1 out]
              }
            }
          }
        }
        n195 = property on="Select Signal to Import" class="MCListbox (strict)"("ItemNames"=string[][] [] ("Item Names"), "Value"=i32[] [] ("Select Signal to Import")) -> ()  [unwired: 2 in, 2 out]
        n196 = Close Reference(reference=w545, error in (no error)=w544) -> (error out=w534:errorcluster)
      }
      frame "SEND MSG" {
        n197 = call-dynamic "Get Message Window Ref.vi"("reference in"=w571, "error in (no error)"=w570) -> ("Msg Win Ref"=w567:refnum<vi>, "error out"=w569:errorcluster)  [unwired: 15 in, 1 out]
        n198 = property class="VI"(reference=w567, error in=w569) -> (reference out=w573:refnum<vi>, error out=w572:errorcluster, "Front Panel.Open"=w574:bool)
        n199 = case shown="False" w574 {
          tunnel: [w588 w592] -> w576
          tunnel: w572 -> [w583 w592]
          tunnel: w573 -> [w585 w591]
          tunnel: [w587 w591] -> w575
          frame False {
            w586 = FALSE ("Wait Until Done")
            n200 = invoke class="VI" method="Run VI"(reference=w585, error in=w583, "Wait until done"=w586, "Auto Dispose Ref"=w586) -> (reference out=w584:refnum<vi>, error out=w582:errorcluster)  [unwired: 1 in, 3 out]
            n201 = invoke class="VI" method="FP.Open"(reference=w584, error in=w582, "Activate"=TRUE, "State"=T2."Standard") -> (reference out=w587:refnum<vi>, error out=w588:errorcluster)  [unwired: 1 in, 3 out]
          }
          frame True {
          }
        }
        n202 = Concatenate Strings("\r\n", w580) -> (w579:string)
        n203 = invoke class="VI" method="Ctrl Val.Set"(reference=w575, error in=w576, "Control Name"="Message", "Value"=w579) -> (error out=w568:errorcluster)  [unwired: 1 in, 4 out]
      }
      frame "CLOSE MSG" {
        n204 = call-dynamic "Get Message Window Ref.vi"("reference in"=w596, "error in (no error)"=w597) -> ("Msg Win Ref"=w594:refnum<vi>, "error out"=w595:errorcluster)  [unwired: 15 in, 1 out]
        n205 = property class="VI"(reference=w594, error in=w595) -> (reference out=w601:refnum<vi>, error out=w602:errorcluster, "Front Panel.Open"=w600:bool)
        n206 = case shown="True" w600 {
          tunnel: [w605 w609] -> w599
          tunnel: w602 -> [w605 w608]
          tunnel: w601 -> [w604 w607]
          tunnel: [w604 w606] -> w598
          frame False {
          }
          frame True {
            n207 = invoke class="VI" method="FP.Close"(reference=w607, error in=w608) -> (reference out=w606:refnum<vi>, error out=w609:errorcluster)  [unwired: 1 in, 1 out]
          }
        }
        n208 = invoke class="VI" method="Abort VI"(reference=w598, error in=w599) -> (error out=w593:errorcluster)  [unwired: 1 in, 2 out]
      }
      frame "---- Miscelleneous ----" {
      }
      frame "unknown", Default {
        n209 = Concatenate Strings("The following state is unrecognized?\n", w614) -> (w613:string)
        n210 = One Button Dialog(message=w613) -> ()  [unwired: 1 in, 1 out]
      }
      frame "Error" {
        n211 = call <vilib>:"General Error Handler.vi"("error in (no error)"=w617) -> ()  [unwired: 10 in, 5 out]
      }
      frame "Next" {
        # "This is an empty case used so the queue does NOT stop if there is an empty string between two valid states!"
      }
      frame "Quit" {
        # "This is the case used to simply exit when this GUI is used as a SubVI!"
        n212 = call-dynamic "Destroy.vi"("reference in"=w622, "error in (no error)"=w623) -> ("error out"=w624:errorcluster)  [unwired: 16 in, 1 out]
      }
    }
    "State Index" <- w18
  }
  "error out" <- w2
  "SubVI Time Data DUP" <- "Time Data IN"
